vi "list_folder-basic.vi"(8 "error in (no error)":errorcluster, 10 "recursive":bool, 11 "path":string) -> (0 "error out":errorcluster, 2 "has_more":bool, 3 "path []":string[](array[string]))   [LabVIEW 2015, in "lv-dropbox.lvlib" / "v2.lvlib"]
uses:
  v2.lvlib
  <vilib>/httpClient/POSTBuffer.vi
  <vilib>/httpClient/LabVIEWHTTPClient.lvlib
  lv-dropbox.lvlib
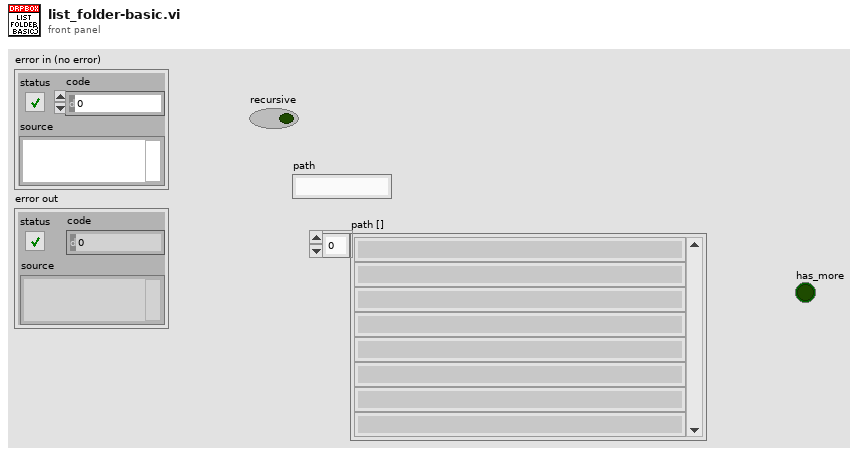
[diagram p1: front panel]
types:
  T1 = cluster{"entries":cluster{".tag":string, "name":string, "path_lower":string, "path_display":string, "id":string}[], "has_more":bool}
  T2 = cluster{"path":string, "recursive":bool, "include_media_info":bool, "include_deleted":bool}
  T3 = typedef "LabVIEWHTTPClient.lvlib/ClientHandle.ctl" = refnum<k1>
  T4 = cluster{".tag":string, "name":string, "path_lower":string, "path_display":string, "id":string}[]
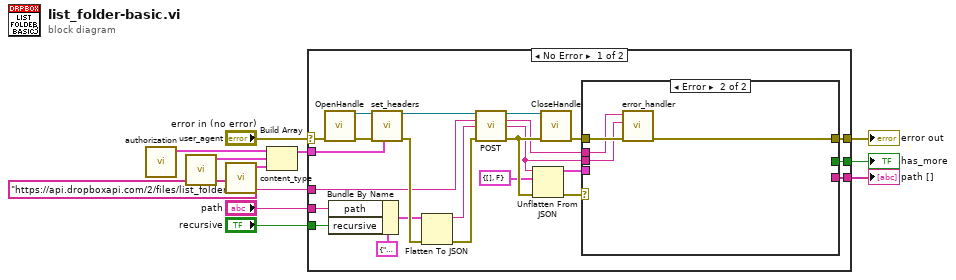
[diagram p0: block diagram]
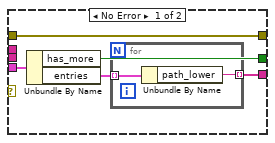
[diagram p2: hidden frame]
diagram:
  n1 = call "authorization.vi"() -> ("header"=w4:cluster{"header":string, "value":string})  [unwired: 11 in]
  n2 = call "user_agent.vi"() -> ("header"=w7:cluster{"header":string, "value":string})  [unwired: 11 in]
  n3 = call "content_type.vi"() -> ("header"=w8:cluster{"header":string, "value":string})  [unwired: 11 in]
  n4 = Build Array(w4, w7, w8) -> (w5:cluster{"header":string, "value":string}[])
  n5 = case shown="No Error" "error in (no error)" {
    selector: "error in (no error)" -> [w20 w47]
    tunnel: [w14 w47] -> w11
    tunnel: "recursive" -> [w32 _]
    tunnel: "path" -> [w31 _]
    tunnel: "https://api.dropboxapi.com/2/files/list_folder" ("url") -> [w25 _]
    tunnel: w5 -> [w21 _]
    tunnel: [w19 _] -> w2
    tunnel: [w18 _] -> w1
    frame No Error {
      n6 = call <vilib>:"OpenHandle.vi"("error in (no error)"=w20) -> ("client handle out"=w24:T3, "error out"=w22:errorcluster)  [unwired: 13 in]
      n7 = Bundle By Name(cluster=T2 {"path"="", "recursive"=FALSE, "include_media_info"=FALSE, "include_deleted"=FALSE}, "path"=w31, "recursive"=w32) -> (w29:T2)
      n8 = call "set_headers.vi"("header_value []"=w21, "error in (no error)"=w22, "client_handle in"=w24) -> ("error out"=w34:errorcluster, "client_handle out"=w23:T3)  [unwired: 7 in]
      n9 = Flatten To JSON(anything=w29, error in (no error)=w34) -> (JSON string=w28:string, 11:w33:errorcluster)  [unwired: 1 in]
      n10 = call-poly <vilib>:"POST.vi"("client handle"=w23, "url"=w25, "buffer"=w28, "error in (no error)"=w33) -> ("client handle out"=w30:T3, "headers"=w13:string, "body"=w12:string, "error out"=w35:errorcluster)  [unwired: 8 in]
      n11 = Unflatten From JSON(JSON string=w12, type and defaults=T1 {"entries"=[], "has_more"=FALSE}, error in (no error)=w35) -> (value=w27:T1, error out=w16:errorcluster)  [unwired: 4 in]
      n12 = call <vilib>:"CloseHandle.vi"("client handle"=w30, "error in (no error)"=w35) -> ("error out"=w15:errorcluster)  [unwired: 13 in]
      n13 = case shown="Error" w16 {
        tunnel: w27 -> [w40 _]
        tunnel: [w38 _] -> w19
        tunnel: [w37 _] -> w18
        tunnel: w15 -> [w36 w46]
        tunnel: [w36 w43] -> w14
        tunnel: w13 -> [_ w45]
        tunnel: w12 -> [_ w44]
        frame No Error {
          n14 = Unbundle By Name(w40) -> ("has_more"=w37:bool, "entries"=w39:T4)
          n15 = for {
            tunnel: w39 -> [w42] mode=indexing
            tunnel: [w41] -> w38 mode=indexing
            n16 = Unbundle By Name(w42) -> ("path_lower"=w41:string)
          }
        }
        frame Error {
          n17 = call "error_handler.vi"("error in (no error)"=w46, "body"=w44, "headers"=w45) -> ("error out"=w43:errorcluster)  [unwired: 8 in]
        }
      }
    }
    frame Error {
    }
  }
  "error out" <- w11
  "path []" <- w2
  "has_more" <- w1
